vi "Ej4.vi"(1 "Temp Scale":bool) -> (0 "Thermometer":dbl(slide) scale=0.0..100.0)   [LabVIEW 2023]
doc: "This VIs measure the output voltage of a simulated temperature sensor in degrees celsius or farenheit depending on the value on the Temp Scale input."
panel:
  # "DegC"
  # "DegF"
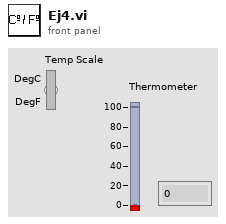
[diagram p1: front panel]
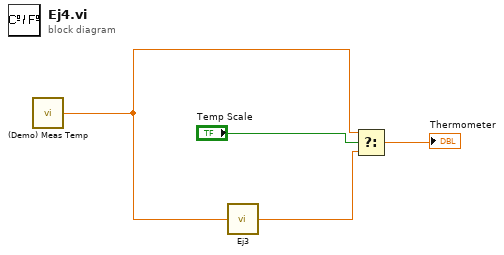
[diagram p0: block diagram]
diagram:
  n1 = call "(Demo) Meas Temp.vi"() -> ("voltage"=w4:dbl)  [unwired: 4 in]
  n2 = call "Ej3.vi"("Deg C"=w4) -> ("Deg F"=w3:dbl)
  n3 = Select(t=w4, s="Temp Scale", f=w3) -> (s? t:f=→"Thermometer":dbl)
